vi "Update Instrument Specifications.vi"(0 "Queue in":refnum<queue>, 1 "Serial Numbers Ref":refnum<vi>, 5 "Instrument Specifications in":T4, 7 "OldVal":T1, 9 "NewVal":T1, 11 "error in (no error)":errorcluster) -> (4 "Queue out":refnum<queue>, 6 "Measurements":T2[](array[typedef]), 8 "Instrument Specifications out":T4, 10 "Serial Numbers":string[](array[string]), 14 "Serial Number Header?":bool, 15 "error out":errorcluster)   [LabVIEW 2026, in "Settings.lvlib"]
uses:
  Settings.lvlib
  Acquisition/Instrument Specifications Configuration.ctl
  Acquisition/Instrument Specifications Cluster Configuration.ctl
  controls/UI/Measurement Role.ctl
  support/Architecture/Message Queue/Message Cluster.ctl
  controls/UI/Measurement Config.ctl
  controls/UI/Measurements Config.ctl
  controls/Messaging Payloads/MSG FetchSensorID Payload.ctl
  Database/Database.lvlib
  Acquisition/Acquisition.lvlib
  support/Architecture/Message Queue/Message Queue.lvlib
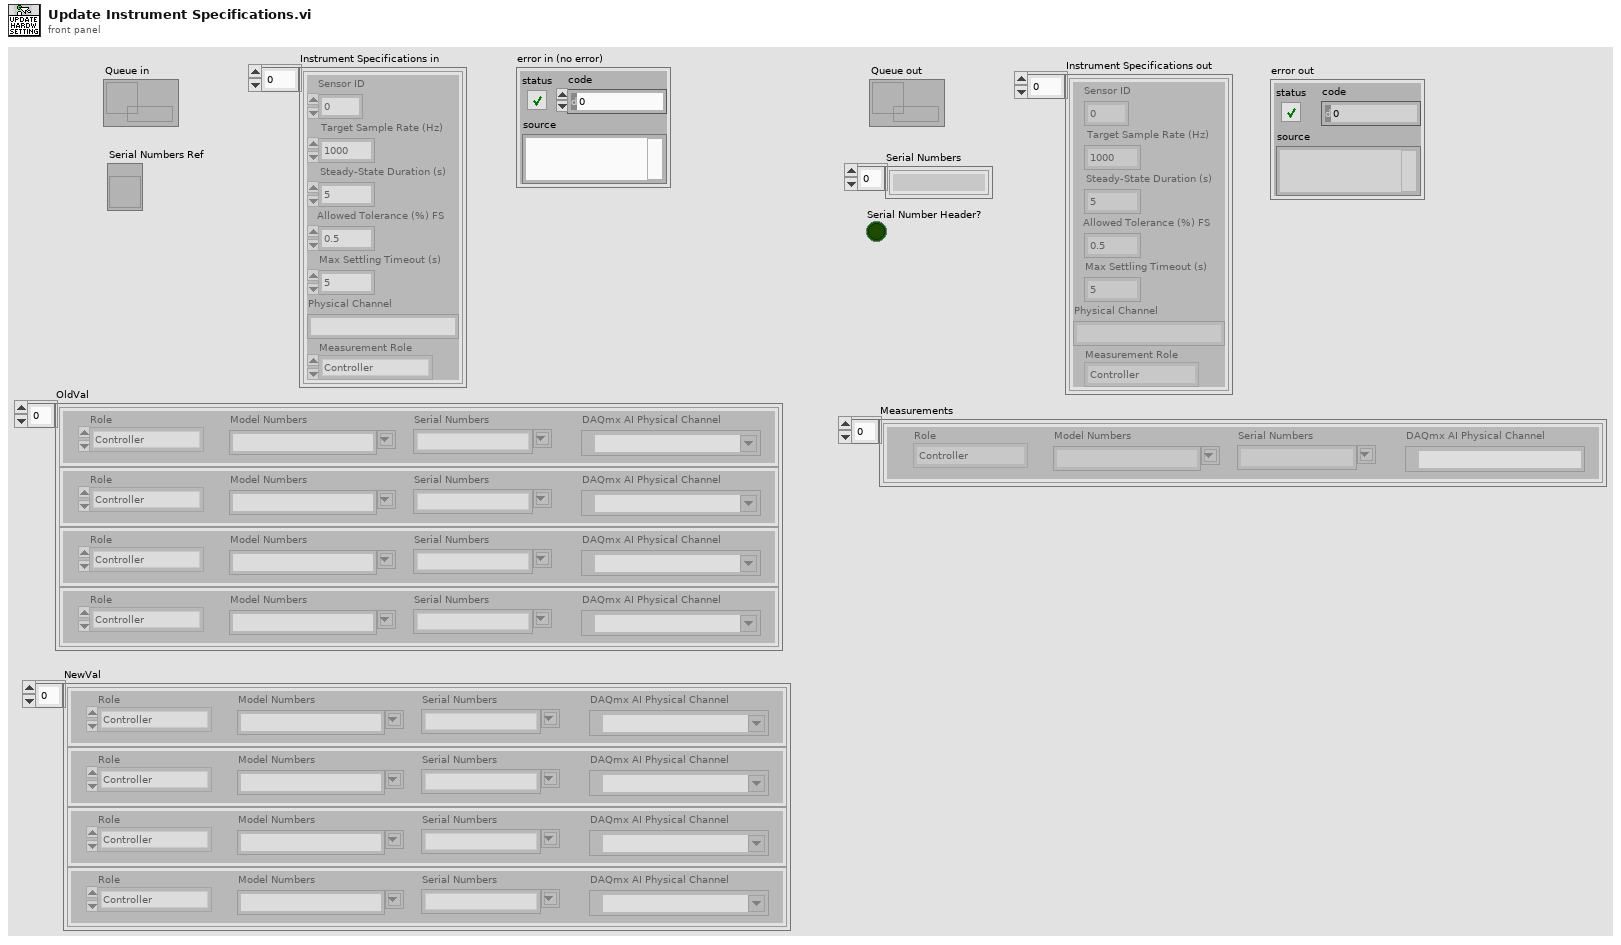
[diagram p1: front panel]
types:
  T1 = typedef "Measurements Config.ctl" = T2[]
  T2 = typedef "Measurement Config.ctl" = cluster{"DAQmx AI Physical Channel":tag, "Serial Numbers":string, "Model Numbers":string, "Role":T3}
  T3 = typedef "Settings.lvlib/Measurement Role.ctl" = enum16{"Controller", "Reference", "UUT", "Disable", "All"}
  T4 = typedef "Acquisition.lvlib/Instrument Specifications Configuration.ctl" = T5[]
  T5 = typedef "Acquisition.lvlib/Instrument Specifications Cluster Configuration.ctl" = cluster{"Sensor ID":i32, "Target Sample Rate (Hz)":dbl, "Steady-State Duration (s)":i32, "Allowed Tolerance (%) FS":dbl, "Max Settling Timeout (s)":i32, "Physical Channel":string, "Measurement Role":T3}
  T6 = typedef "Database.lvlib/MSG FetchSensorID Payload.ctl" = cluster{"SensorID":i32, "Serial Number":string, "Model Number":string}
  T7 = typedef "MSG FetchConfiguration Payload.ctl" = cluster{"Serial Numbers":string[], "Hardware Settings Cluster":T5}
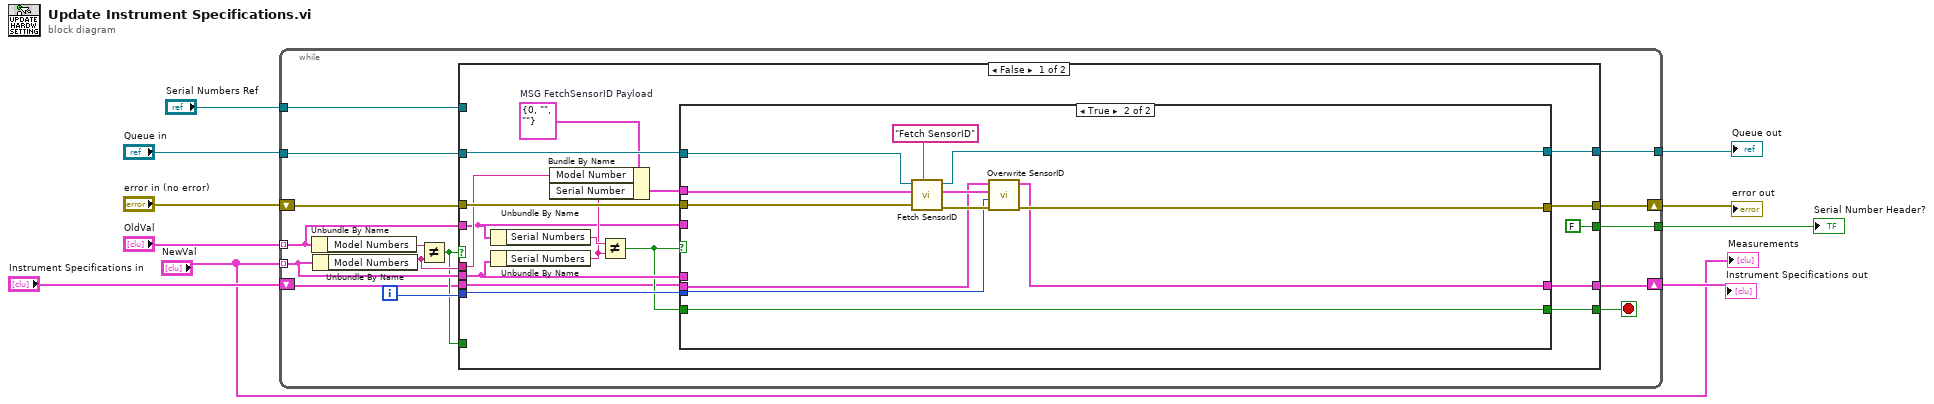
[diagram p0: block diagram]
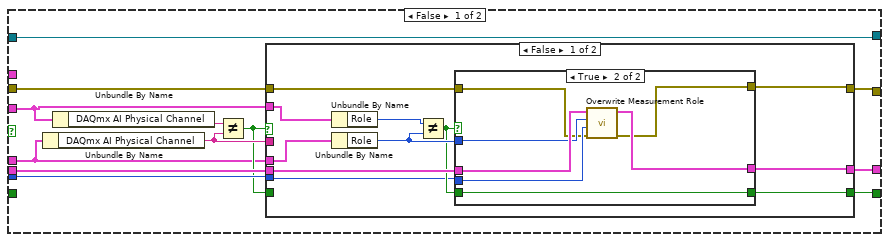
[diagram p2: hidden frame]
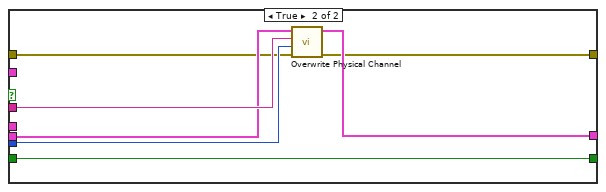
[diagram p4: hidden frame]
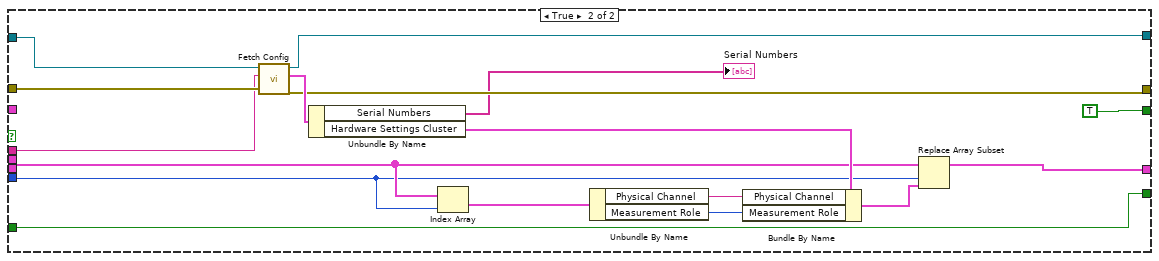
[diagram p5: hidden frame]
diagram:
  n1 = while {
    tunnel: "OldVal" -> [w23] mode=indexing
    tunnel: "NewVal" -> [w17] mode=indexing
    tunnel: "Queue in" -> [w25]
    shift-right: [w22] -> w6
    shift-left: "error in (no error)" -> [w21]
    tunnel: [w20] -> w8
    shift-right: [w19] -> w9
    shift-left: "Instrument Specifications in" -> [w11]
    tunnel: "Serial Numbers Ref" -> [w15]
    tunnel: [w14] -> w1
    i -> [w18]
    stop <- w12 stop-if-true
    n2 = Unbundle By Name(w23) -> ("Model Numbers"=w24:string)
    n3 = Unbundle By Name(w17) -> ("Model Numbers"=w16:string)
    n4 = Not Equal?(x=w24, y=w16) -> (x != y?=w13:bool)
    n5 = case shown="False" w13 {
      tunnel: w25 -> [w41 w111]
      tunnel: w23 -> [w31 _]
      tunnel: [w37 w102] -> w19
      tunnel: w21 -> [w40 w110]
      tunnel: [w36 w106] -> w22
      tunnel: [w39 w108] -> w20
      tunnel: w18 -> [w38 w99]
      tunnel: w11 -> [w26 w100]
      tunnel: w17 -> [w30 _]
      tunnel: w16 -> [w33 w107]
      tunnel: w15 -> [_ _]
      tunnel: [FALSE TRUE] -> w14
      tunnel: [w27 w104] -> w12
      tunnel: w13 -> [_ w104]
      frame False {
        w35 = T6 {"SensorID"=0, "Serial Number"="", "Model Number"=""}  # MSG FetchSensorID Payload
        n6 = Unbundle By Name(w31) -> ("Serial Numbers"=w42:string)
        n7 = Unbundle By Name(w30) -> ("Serial Numbers"=w32:string)
        n8 = Bundle By Name(cluster=w35, "Model Number"=w33, "Serial Number"=w32) -> (w34:T6)
        n9 = Not Equal?(x=w42, y=w32) -> (x != y?=w28:bool)
        n10 = case shown="True" w28 {
          tunnel: w41 -> [w47 w94]
          tunnel: w40 -> [w49 w93]
          tunnel: [w48 w89] -> w36
          tunnel: [w47 w91] -> w39
          tunnel: w38 -> [w52 w88]
          tunnel: w26 -> [w51 w83]
          tunnel: [w50 w87] -> w37
          tunnel: w34 -> [_ w85]
          tunnel: w31 -> [w44 _]
          tunnel: w30 -> [w43 _]
          tunnel: w28 -> [_ w84]
          tunnel: [w46 w84] -> w27
          frame False {
            n11 = Unbundle By Name(w43) -> ("DAQmx AI Physical Channel"=w53:tag)
            n12 = Unbundle By Name(w44) -> ("DAQmx AI Physical Channel"=w54:tag)
            n13 = Not Equal?(x=w54, y=w53) -> (x != y?=w45:bool)
            n14 = case shown="False" w45 {
              tunnel: w53 -> [_ w81]
              tunnel: w52 -> [w55 w82]
              tunnel: w51 -> [w62 w80]
              tunnel: [w58 w79] -> w50
              tunnel: w49 -> [w60 w78]
              tunnel: [w59 w77] -> w48
              tunnel: w45 -> [_ w76]
              tunnel: [w56 w76] -> w46
              tunnel: w44 -> [w64 _]
              tunnel: w43 -> [w63 _]
              frame False {
                n15 = Unbundle By Name(w64) -> ("Role"=w65:T3)
                n16 = Unbundle By Name(w63) -> ("Role"=w61:T3)
                n17 = Not Equal?(x=w65, y=w61) -> (x != y?=w57:bool)
                n18 = case shown="True" w57 {
                  tunnel: w62 -> [w67 w75]
                  tunnel: w61 -> [_ w74]
                  tunnel: w60 -> [w68 w70]
                  tunnel: [w68 w69] -> w59
                  tunnel: [w67 w73] -> w58
                  tunnel: w57 -> [w66 w72]
                  tunnel: [w66 w72] -> w56
                  tunnel: w55 -> [_ w71]
                  frame False {
                  }
                  frame True {
                    n19 = call "Overwrite Measurement Role.vi"("Instrument Specifications in"=w75, "Measurement Role"=w74, "Index"=w71, "error in (no error)"=w70) -> ("Instrument Specifications out"=w73:T4, "error out"=w69:errorcluster)  [unwired: 5 in]
                  }
                }
              }
              frame True {
                n20 = call "Overwrite Physical Channel.vi"("error in (no error)"=w78, "Index"=w82, "DAQmx Physical Channel"=w81, "Instrument Specifications in"=w80) -> ("error out"=w77:errorcluster, "Instrument Specifications out"=w79:T4)  [unwired: 6 in]
              }
            }
          }
          frame True {
            n21 = call "Fetch SensorID.vi"("Message"="Fetch SensorID", "error in (no error)"=w93, "MSG FetchSensorID Payload in"=w85, "Database in"=w94) -> ("error out"=w90:errorcluster, "MSG FetchSensorID Payload out"=w86:T6, "Database out"=w91:refnum<queue>)  [unwired: 5 in]
            n22 = call "Overwrite SensorID.vi"("error in (no error)"=w90, "Index"=w88, "MSG FetchSensorID Payload"=w86, "Instrument Specifications in"=w83) -> ("error out"=w89:errorcluster, "Instrument Specifications out"=w87:T4)  [unwired: 6 in]
          }
        }
      }
      frame True {
        n23 = call "Fetch Config.vi"("error in (no error)"=w110, "ModelNumber"=w107, "Database in"=w111) -> ("error out"=w106:errorcluster, "Model Details Payload"=w109:T7, "Database out"=w108:refnum<queue>)  [unwired: 6 in]
        n24 = Unbundle By Name(w109) -> ("Serial Numbers"=→"Serial Numbers":string[], "Hardware Settings Cluster"=w101:T5)
        n25 = Index Array(array=w100, index=w99) -> (element=w98:T5)
        n26 = Unbundle By Name(w98) -> ("Physical Channel"=w97:string, "Measurement Role"=w96:T3)
        n27 = Bundle By Name(cluster=w101, "Physical Channel"=w97, "Measurement Role"=w96) -> (w95:T5)
        n28 = Replace Array Subset(array=w100, new element=w95, index=w99) -> (w102:T4)
      }
    }
  }
  "Instrument Specifications out" <- w9
  "Queue out" <- w8
  "error out" <- w6
  "Serial Number Header?" <- w1
  "Measurements" <- "NewVal"
